vi "PBLV_Example1.vi"() -> ()   [LabVIEW 2012]
panel:
  in  "PB Inst 2":T1={"Instruct Data"=0, "Op Code"=6, "Flags"=[FALSE, FALSE, FALSE, FALSE, FALSE, FALSE, FALSE, FALSE, FALSE, FALSE, FALSE, FALSE, FALSE, FALSE, FALSE, FALSE, FALSE, FALSE, FALSE, FALSE, FALSE, FALSE, FALSE, FALSE], "Comments"="", "Time (s)"=0.1} {"Time (s)" format="%.3p"; "Op Code" items=["Continue", "Stop", "Loop", "End Loop", "JSR", "RTS", "Branch", "Long Delay", "Wait"]}
  in  "PB Inst 1":T1={"Instruct Data"=0, "Op Code"=0, "Flags"=[FALSE, FALSE, FALSE, FALSE, FALSE, FALSE, FALSE, FALSE, FALSE, FALSE, FALSE, FALSE, FALSE, FALSE, FALSE, FALSE, FALSE, FALSE, FALSE, FALSE, FALSE, FALSE, FALSE, FALSE], "Comments"="", "Time (s)"=0.1} {"Time (s)" format="%.3p"; "Op Code" items=["Continue", "Stop", "Loop", "End Loop", "JSR", "RTS", "Branch", "Long Delay", "Wait"]}
  in  "PB Inst 0":T1={"Instruct Data"=0, "Op Code"=0, "Flags"=[TRUE, FALSE, FALSE, FALSE, FALSE, FALSE, FALSE, FALSE, FALSE, FALSE, FALSE, FALSE, FALSE, FALSE, FALSE, FALSE, FALSE, FALSE, FALSE, FALSE, FALSE, FALSE, FALSE, FALSE], "Comments"="", "Time (s)"=0.2} {"Time (s)" format="%.3p"; "Op Code" items=["Continue", "Stop", "Loop", "End Loop", "JSR", "RTS", "Branch", "Long Delay", "Wait"]}
  in  "Location of spinapi.dll":path=path "C:/SpinCore/SpinAPI/dll/spinapi.dll"
  in  "start/restart":bool
  in  "load":bool
  in  "stop":bool
  in  "clock_freq (MHz)":dbl=100.0
  # "SpinCore PulseBlaster LabVIEW Extensions\nExample 1\nSpinCore Technologies, Inc.\nwww.spincore.com"
  # "Caution:    \n            After pressing \n            STOP, all output bits may maintain their final state."
  # "1"
  # "2"
  # "3"
  # "4"
  # "5"
  # "6"
  # "7"
  # "8"
  # "9"
  # "10"
  # "11"
  # "12"
  # "13"
  # "14"
  # "15"
  # "16"
  # "17"
  # "18"
  # "19"
  # "20"
  # "21"
  # "22"
  # "23"
  # "24"
  # "1"
  # "2"
  # "3"
  # "4"
  # "5"
  # "6"
  # "7"
  # "8"
  # "9"
  # "10"
  # "11"
  # "12"
  # "13"
  # "14"
  # "15"
  # "16"
  # "17"
  # "18"
  # "19"
  # "20"
  # "21"
  # "22"
  # "23"
  # "24"
  # "1"
  # "2"
  # "3"
  # "4"
  # "5"
  # "6"
  # "7"
  # "8"
  # "9"
  # "10"
  # "11"
  # "12"
  # "13"
  # "14"
  # "15"
  # "16"
  # "17"
  # "18"
  # "19"
  # "20"
  # "21"
  # "22"
  # "23"
  # "24"
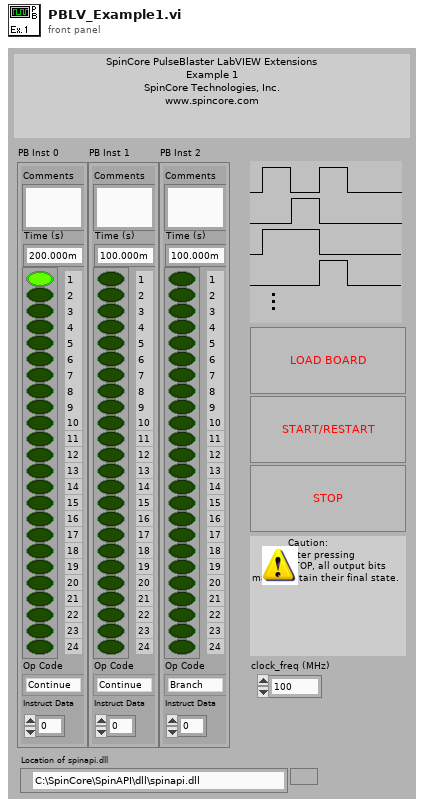
[diagram p1: front panel]
types:
  T1 = cluster{"Instruct Data":i32, "Op Code":i32, "Flags":bool[], "Comments":string, "Time (s)":dbl}
  T2 = enum16{"Pulse Program", "Frequency Registers", "TX Phase Registers", "RX Phase Registers"}
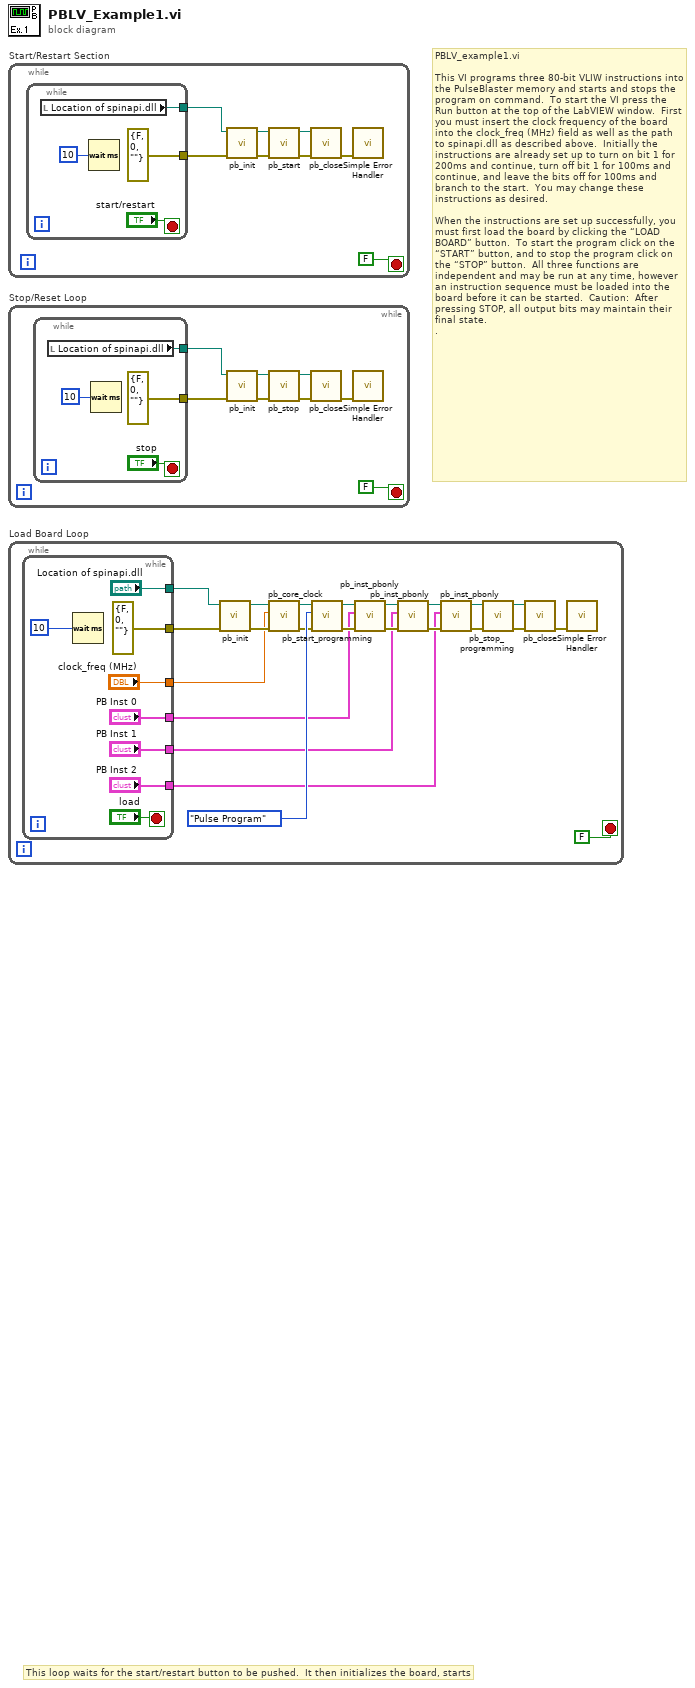
[diagram p0: block diagram]
diagram:
  # "PBLV_example1.vi\n\nThis VI programs three 80-bit VLIW instructions into the PulseBlaster memory and starts and stops the program on command.  To start the VI press the Run button at the top of the LabVIEW window.  First you must insert the clock frequency of the board into the clock_freq (MHz) field as well as the path to spinapi.dll as described above.  Initially the instructions are already set up to turn on bit 1 for 200ms and continue, turn off bit 1 for 100ms and continue, and leave the bits off for 100ms and branch to the start.  You may change these instructions as desired. \n \nWhen the instructions are set up successfully, you must first load the board by clicking the “LOAD BOARD” button.  To start the program click on the “START” button, and to stop the program click on the “STOP” button.  All three functions are independent and may be run at any time, however an instruction sequence must be loaded into the board before it can be started.  Caution:  After pressing STOP, all output bits may maintain their final state.\n."
  # "This loop waits for the start/restart button to be pushed.  It then initializes the board, starts"
  n1 = while "Start/Restart Section" {
    stop <- FALSE stop-if-true
    n2 = while {
      tunnel: [errorcluster {"status"=FALSE, "code"=0, "source"=""} ("error in (no error)")] -> w7
      tunnel: [w9] -> w1
      stop <- "start/restart" stop-if-true
      n3 = local read "Location of spinapi.dll"() -> (w9:path)
      n4 = Wait (ms)(milliseconds to wait=u32 10) -> ()  [unwired: 1 out]
    }
    n5 = call "pb_init.vi"("error in (no error)"=w7, "path in"=w1) -> ("error out"=w5:errorcluster, "path out"=w6:path)  [unwired: 1 in, 7 out]
    n6 = call "pb_start.vi"("error in (no error)"=w5, "path in"=w6) -> ("error out"=w3:errorcluster, "path out"=w4:path)  [unwired: 1 in, 7 out]
    n7 = call "pb_close.vi"("error in (no error)"=w3, "path in"=w4) -> ("error out"=w2:errorcluster)  [unwired: 9 out]
    n8 = call <vilib>:"Simple Error Handler.vi"("error in (no error)"=w2) -> ()  [unwired: 1 in, 8 out]
  }
  n9 = while "Stop/Reset Loop" {
    stop <- FALSE stop-if-true
    n10 = while {
      tunnel: [errorcluster {"status"=FALSE, "code"=0, "source"=""} ("error in (no error)")] -> w19
      tunnel: [w21] -> w13
      stop <- "stop" stop-if-true
      n11 = local read "Location of spinapi.dll"() -> (w21:path)
      n12 = Wait (ms)(milliseconds to wait=u32 10) -> ()  [unwired: 1 out]
    }
    n13 = call "pb_init.vi"("error in (no error)"=w19, "path in"=w13) -> ("error out"=w17:errorcluster, "path out"=w18:path)  [unwired: 1 in, 7 out]
    n14 = call "pb_stop.vi"("error in (no error)"=w17, "path in"=w18) -> ("error out"=w15:errorcluster, "path out"=w16:path)  [unwired: 8 out]
    n15 = call "pb_close.vi"("error in (no error)"=w15, "path in"=w16) -> ("error out"=w14:errorcluster)  [unwired: 9 out]
    n16 = call <vilib>:"Simple Error Handler.vi"("error in (no error)"=w14) -> ()  [unwired: 1 in, 8 out]
  }
  n17 = while "Load Board Loop" {
    stop <- FALSE stop-if-true
    n18 = while {
      tunnel: [errorcluster {"status"=FALSE, "code"=0, "source"=""} ("error in (no error)")] -> w44
      tunnel: ["PB Inst 0"] -> w33
      tunnel: ["PB Inst 1"] -> w32
      tunnel: ["PB Inst 2"] -> w31
      tunnel: ["Location of spinapi.dll"] -> w26
      tunnel: ["clock_freq (MHz)"] -> w25
      stop <- "load" stop-if-true
      n19 = Wait (ms)(milliseconds to wait=u32 10) -> ()  [unwired: 1 out]
    }
    n20 = call "pb_init.vi"("error in (no error)"=w44, "path in"=w26) -> ("error out"=w28:errorcluster, "path out"=w30:path)  [unwired: 2 in, 6 out]
    n21 = call "pb_core_clock.vi"("error in (no error)"=w28, "clock_freq (MHz)"=w25, "path in"=w30) -> ("error out"=w27:errorcluster, "path out"=w29:path)  [unwired: 7 in]
    n22 = call "pb_start_programming.vi"("error in (no error)"=w27, "Device"=T2."Pulse Program", "path in"=w29) -> ("error out"=w41:errorcluster, "path out"=w42:path)  [unwired: 1 in, 6 out]
    n23 = call "pb_inst_pbonly.vi"("error in (no error)"=w41, "PB Instruction"=w33, "path in"=w42) -> ("error out"=w40:errorcluster, "path out"=w47:path)  [unwired: 2 in, 5 out]
    n24 = call "pb_inst_pbonly.vi"("error in (no error)"=w40, "PB Instruction"=w32, "path in"=w47) -> ("error out"=w39:errorcluster, "path out"=w46:path)  [unwired: 2 in, 5 out]
    n25 = call "pb_inst_pbonly.vi"("error in (no error)"=w39, "PB Instruction"=w31, "path in"=w46) -> ("error out"=w37:errorcluster, "path out"=w38:path)  [unwired: 2 in, 5 out]
    n26 = call "pb_stop_programming.vi"("error in (no error)"=w37, "path in"=w38) -> ("error out"=w35:errorcluster, "path out"=w36:path)  [unwired: 1 in, 7 out]
    n27 = call "pb_close.vi"("error in (no error)"=w35, "path in"=w36) -> ("error out"=w34:errorcluster)  [unwired: 9 out]
    n28 = call <vilib>:"Simple Error Handler.vi"("error in (no error)"=w34) -> ()  [unwired: 1 in, 8 out]
  }
